vi "Init.vi"(8 "error in (no error)":errorcluster, 11 "Control VI":T1) -> (0 "error out":errorcluster, 3 "FormulaLV App out":refnum<class "FormulaG App.lvclass">)   [LabVIEW 2020, in "FormulaG.lvlib" / "FormulaG App.lvclass"]
uses:
  FormulaG App.lvclass
  FormulaLV-Common/Control VI.ctl
  FormulaG App.lvclass/FormulaG App.ctl
  FormulaLV-Common/FormulaG-Common.lvlib
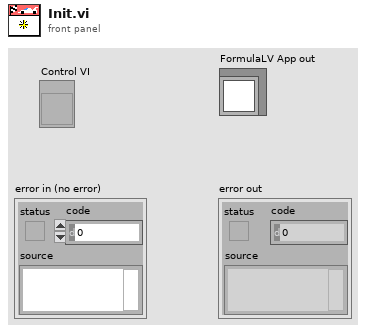
[diagram p1: front panel]
types:
  T1 = typedef "FormulaG-Common.lvlib/Control VI.ctl" = refnum<vi>
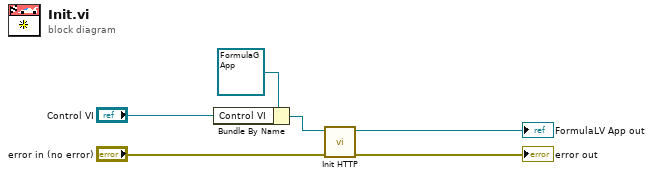
[diagram p0: block diagram]
diagram:
  n1 = Bundle By Name(cluster=refnum<class "FormulaG App.lvclass"> refnum ("FormulaLV App in"), "Control VI"="Control VI") -> (w2:refnum<class "FormulaG App.lvclass">)
  n2 = call "Init HTTP.vi"("error in (no error)"="error in (no error)", "FormulaLV App in"=w2) -> ("error out"=→"error out":errorcluster, "FormulaLV App out"=→"FormulaLV App out":refnum<class "FormulaG App.lvclass">)  [unwired: 8 in]
